vi "Berekenen-a.vi"(6 "K":dbl, 9 "Ti":dbl, 10 "Td":dbl, 11 "T":dbl) -> (2 "A":dbl)   [LabVIEW 2021]
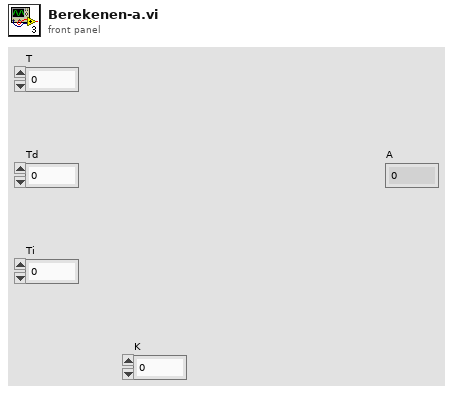
[diagram p1: front panel]
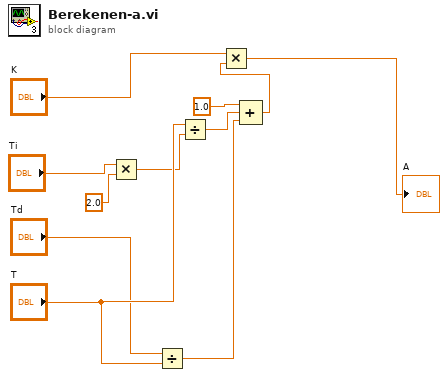
[diagram p0: block diagram]
diagram:
  n1 = Multiply(x="Ti", y=2.0) -> (x*y=w5:dbl)
  n2 = Divide(x="Td", y="T") -> (x/y=w8:dbl)
  n3 = Divide(x="T", y=w5) -> (x/y=w9:dbl)
  n4 = Compound Arithmetic op=ADD(1.0 ("value"), w9, w8) -> (w11:dbl)
  n5 = Multiply(x="K", y=w11) -> (x*y=→"A":dbl)
